vi "All_Combined_final_opt_save_file_P4.vi"() -> ()   [LabVIEW 2018]
uses:
  <vilib>/LabVIEW Interface for Arduino/Type Defs/Board Type.ctl
  Controls created/Control 3.ctl
  Controls created/Control 4.ctl
  <vilib>/LabVIEW Interface for Arduino/Type Defs/Connection Type.ctl
  <instrlib>/LeCroy Wave Series/Public/Data/Read Single Waveform.vi
  <vilib>/Utility/file.llb/Write Delimited Spreadsheet (DBL).vi
  <vilib>/LabVIEW Interface for Arduino/LabVIEW Interface for Arduino.lvlib
  <instrlib>/Siglent SDG X Series/Siglent SDG X Series.lvlib
  <instrlib>/LeCroy Wave Series/LeCroy Wave Series.lvlib
panel:
  in  "Tab Control":enum32{"Page 1", "Page 2", "Page 3"}(tab)
  in  "VISA resource":refnum<visa-resource-name>
  in  "Board Type (Uno)":T1
  in  "Steps for 1 rotation(1600steps)":i16=1600
  in  "Set Speed (Steps/s)":i16=1200 min=0 max=3000 step=50
  out "Steps Remaining? 2":bool
  in  "#Steps":i16
  out "Step Angle":dbl
  in  "Baud Rate":u32=9600
  out "Iteration #":i32
  out "Steps Remaining?":bool
  in  "Total translation distance(in mm)":i16
  out "Error":errorcluster
  in  "#Steps":dbl
  in  "Arbitray Movement":bool
  in  "Stop":bool
  out "Moving?":bool
  out "stop motion":bool
  in  "MOTION":bool
  in  "?":i8(slide) step=2 scale=0.0..2.0
  in  "OK Button":bool
  out "# steps moved":i32
  out "Scan_time":dbl
  out "daq_time":dbl
  out "appended array":dbl[](array[numeric])
  in  "VISA Refnum in":refnum<visa-resource-name>="USB0::0xF4EC::0xEE38::SDG2XCAD2R3765::INSTR"
  in  "Channel (1:Channel 1)":i32(ring)=1 items=["Channel 1"=1, "Channel 2"=2]
  in  "Enable Output (T: Enable)":bool=TRUE
  in  "Amplitude (1.0 Vpp)":dbl=20.0 format="%#.3f"
  in  "Frequency (1000 Hz)":T2=1500000.0 format="%#.6g"
  in  "DC Offset (0.00 V) in":dbl
  in  "Waveform Function (0: Sine) in":u16(ring) items=["Sine", "Square", "Ramp", "DC", "Pulse", "Arb"]
  in  "Phase (0.0 degrees)":dbl=0.002 min=-360.0 max=360.0 format="%#.1g"
  in  "Fall (20 ns)":dbl=8.4e-09 format="%#.3g"
  in  "Duty (20%)":dbl=4.32 min=0.0001 max=100.0 format="%.4g"
  in  "Delay (0.00 s)":dbl min=-1000000.0 max=1000000.0
  in  "Rise (20 ns)":dbl=1.04e-08 format="%#.3g"
  in  "True To \ngenerate\n pulse":T3=TRUE
  out "VISA resource name out":refnum<visa-resource-name>
  out "error out":errorcluster
  out "Output Filename":path
  out "error out 2":errorcluster
  in  "format string":string="Channel: %g \nWavetype: %g \nAMP: %gV\nFreq: %gHz \nRiseTime: %gs \nFallTime: %gs \nDutyCycle: %g"
  out "Output Directory":path
  in  "File Directory":path=path "E:/Ankur/Labview/Automation/Data/Exp1"
  in  "Filename":string
  out "Oscilloscope\n Runnning":bool
  in  "stop":bool
  out "Waveform Data":waveform(dbl)(graph)
  in  "Timeout (10000 ms)":u32=10000
  in  "Source (0: Channel 1)":u16(ring) items=["Channel 1", "Channel 2", "Channel 3", "Channel 4", "Memory 1", "Memory 2", "Memory 3", "Memory 4", "Function 1", "Function 2", "Function 3", "Function 4", "Function 5", "Function 6", "Function 7", "Function 8"]
  in  "Perform Auto Setup?":bool
  in  "Reset Scope?":bool
  in  "VISA resource name":refnum<visa-resource-name>="LecroyHDO4024-1"
  in  "Save Files in Directory (In Oscilloscope)":string="D:\\Automation\\Data"
  in  "Filename":string="Title"
  in  "Path to save DATA":path=path "E:/Ankur/Labview/Automation/Files/Oscdata"
  out "Saved filename":string
  in  "Save File locally":bool
  # "For Rotational motion"
  # "For Translational Motion"
  # "For Translational motion"
  # "OFF"
  # "ON"
  # "Yes"
  # "No"
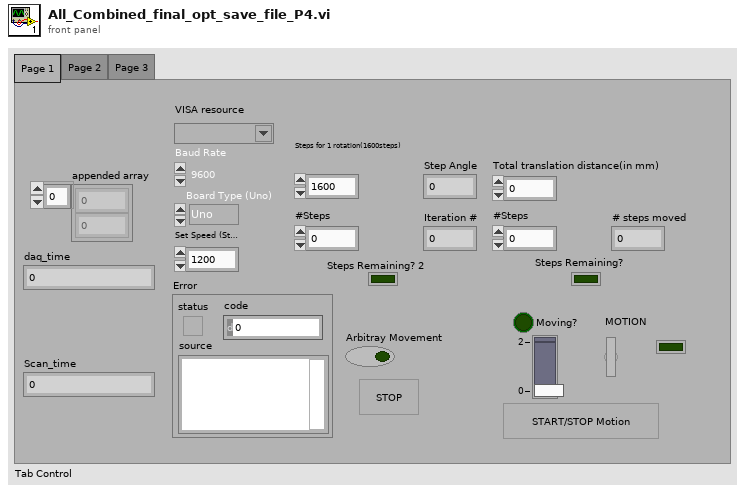
[diagram p1: front panel]
types:
  T1 = typedef "LabVIEW Interface for Arduino.lvlib/Board Type.ctl" = enum16{"Uno", "Dimuelanove w/Atmega 328", "Mega 2560"}
  T2 = typedef "Control 3.ctl" = dbl
  T3 = typedef "Control 4.ctl" = bool
  T4 = typedef "LabVIEW Interface for Arduino.lvlib/Connection Type.ctl" = enum8{"USB / Serial", "XBEE", "BlueSmirf (Bluetooth)"}
  T5 = typedef "LabVIEW Interface for Arduino.lvlib/Arduino Resource.ctl" = cluster{"VISA resource":refnum<visa-resource-name>, "Board Type":T1, "Connection Type":enum8{"USB / Serial"}, "Bytes Per Packet (15)":u8}
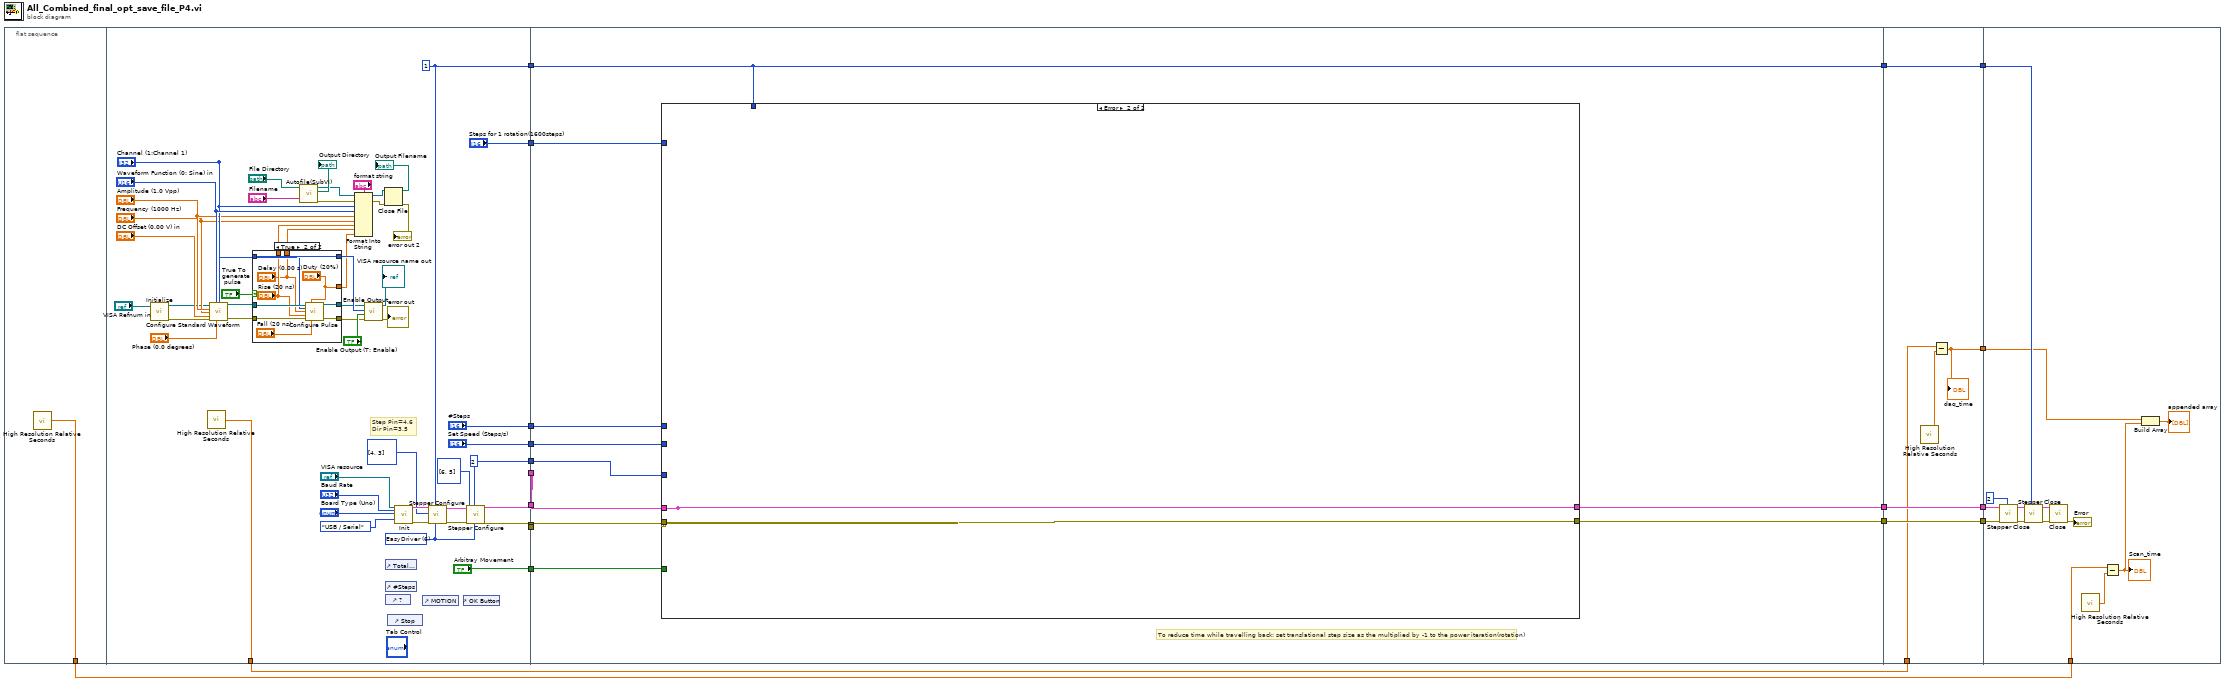
[diagram p0: block diagram]
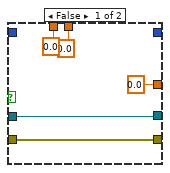
[diagram p2: hidden frame]
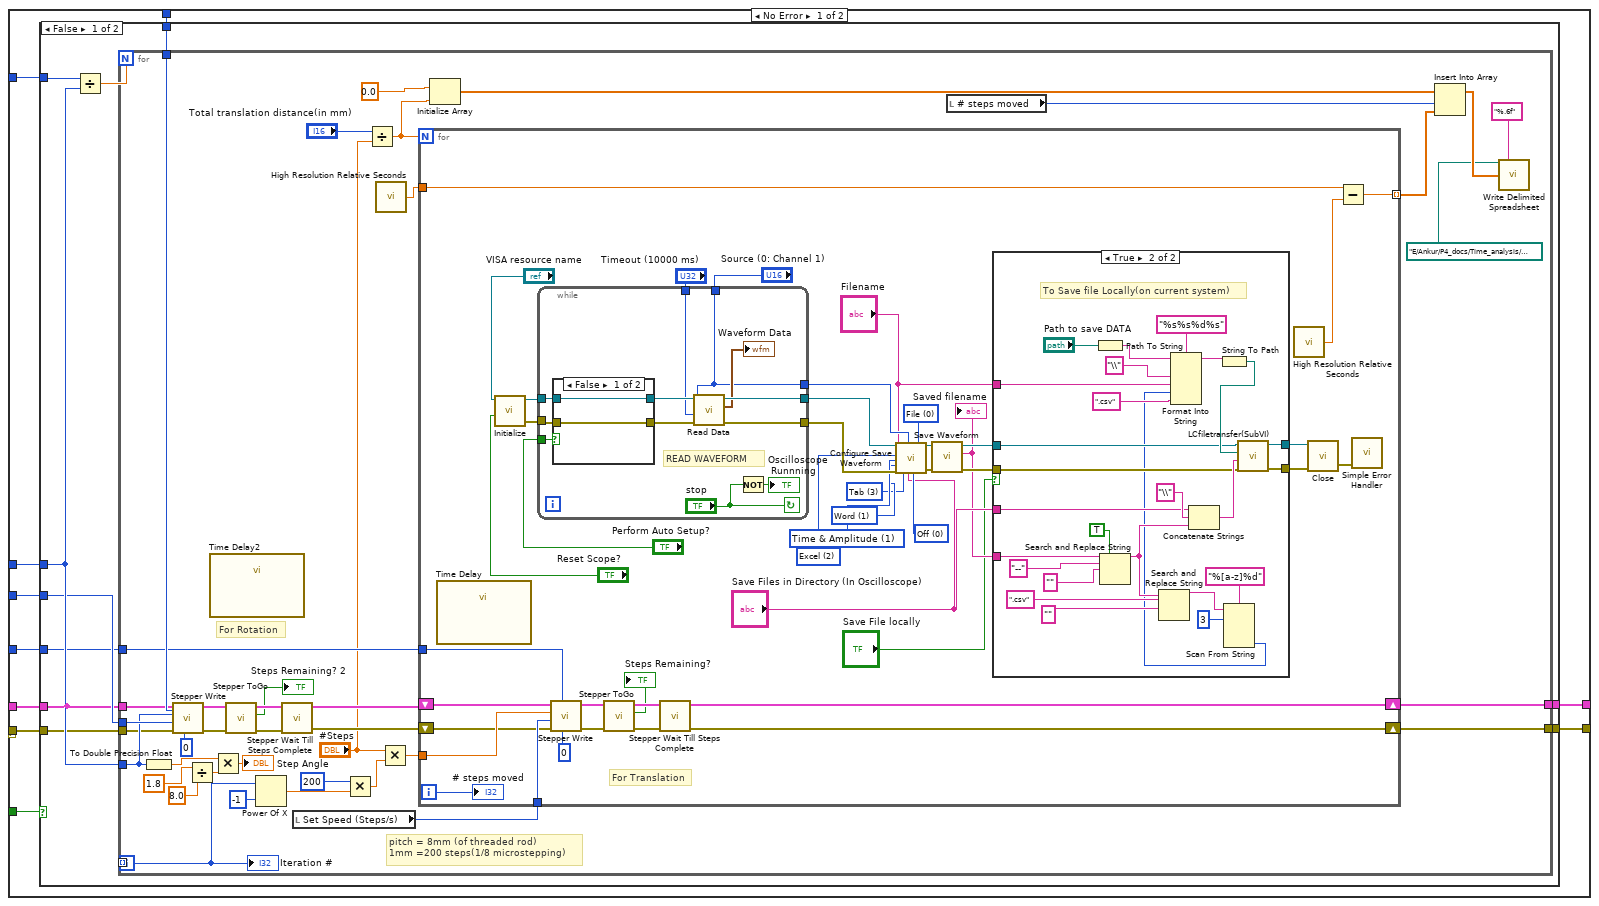
[diagram p3: hidden frame]
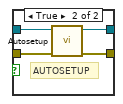
[diagram p5: hidden frame]
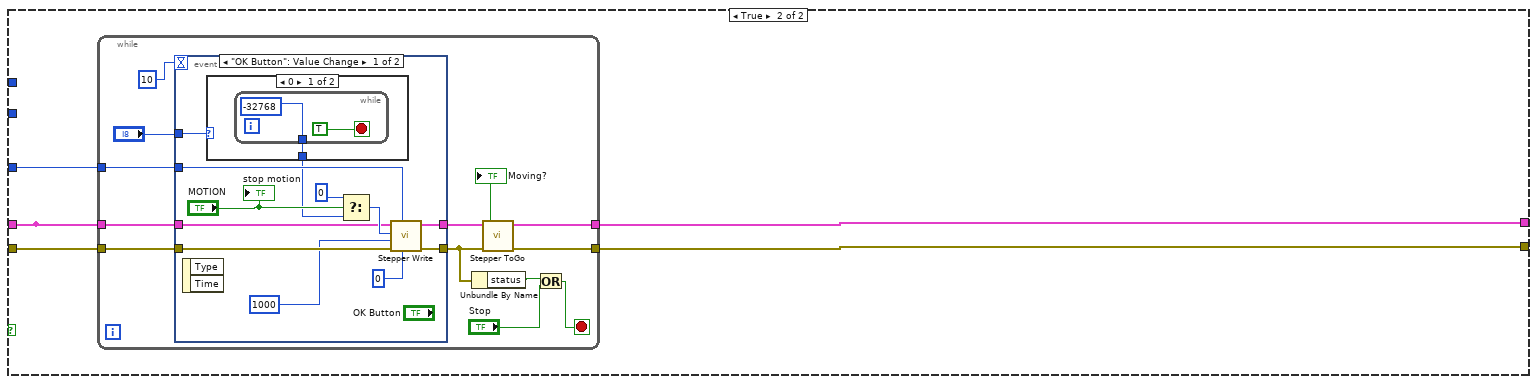
[diagram p6: hidden frame]
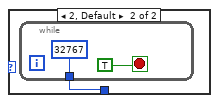
[diagram p7: hidden frame]
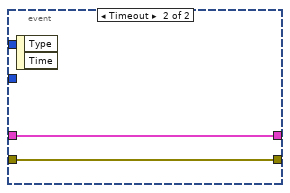
[diagram p8: hidden frame]
diagram:
  n1 = flat-sequence {
    tunnel: [w18] -> w2
    tunnel: [w27] -> w14
    tunnel: [w26] -> w13
    tunnel: [w25] -> w12
    tunnel: [w20] -> w11
    tunnel: ["Arbitray Movement"] -> w10
    tunnel: ["Set Speed (Steps/s)"] -> w9
    tunnel: ["Steps for 1 rotation(1600steps)"] -> w8
    tunnel: ["#Steps"] -> w7
    tunnel: [w19] -> w6
    tunnel: [w89] -> w17
    tunnel: [w92] -> w16
    tunnel: [w91] -> w15
    tunnel: w14 -> [w90]
    tunnel: w13 -> [w89]
    tunnel: w12 -> [w88]
    tunnel: w11 -> [w87]
    tunnel: w10 -> [w86]
    tunnel: w9 -> [w85]
    tunnel: w8 -> [w84]
    tunnel: w7 -> [w83]
    tunnel: w17 -> [w288]
    tunnel: w16 -> [w287]
    tunnel: w15 -> [w286]
    tunnel: w6 -> [w284]
    tunnel: [w288] -> w5
    tunnel: [w287] -> w4
    tunnel: [w286] -> w3
    tunnel: [w283] -> w1
    tunnel: w5 -> [w294]
    tunnel: w4 -> [w296]
    tunnel: w3 -> [w295]
    tunnel: w2 -> [w292]
    tunnel: w1 -> [w291]
    frame #0 {
      n2 = call <vilib>:"High Resolution Relative Seconds.vi"() -> ("relative seconds"=w18:dbl)
    }
    frame #1 {
      w27 = u8 2 ("Stepper #")
      w26 = u8 1 ("Stepper #")
      w31 = u8 6 items=["2 Wire (Pulse & Direction)"=1, "2 Wire"=2, "4 Wire"=4, "EasyDriver"=6, "AF Motor Shield (Stepper 1 & 2 Only)"=5] ("Control Method")
      # "Step Pin=4,6\nDir Pin=3,5"
      n3 = call <instrlib>:"Initialize.vi"("VISA resource name"="VISA Refnum in") -> ("error out"=w44:errorcluster, "VISA resource name out"=w43:refnum<visa-resource-name>)  [unwired: 9 in]
      n4 = call <vilib>:"High Resolution Relative Seconds.vi"() -> ("relative seconds"=w19:dbl)
      n5 = call <instrlib>:"Configure Standard Waveform.vi"("VISA resource name"=w43, "Waveform Function (0: Sine)"="Waveform Function (0: Sine) in", "Channel (1:Channel 1)"="Channel (1:Channel 1)", "Amplitude (1.0 Vpp)"="Amplitude (1.0 Vpp)", "Frequency (1000 Hz)"="Frequency (1000 Hz)", "DC Offset (0.00 V)"="DC Offset (0.00 V) in", "error in (no error)"=w44, "Phase (0.0 degrees)"="Phase (0.0 degrees)") -> ("VISA resource name out"=w48:refnum<visa-resource-name>, "error out"=w45:errorcluster)  [unwired: 6 in]
      n6 = case shown="True" "True To \ngenerate\n pulse" {
        tunnel: [w73 w81] -> w39
        tunnel: [w72 w80] -> w40
        tunnel: w48 -> [w73 w79]
        tunnel: w45 -> [w72 w78]
        tunnel: "Channel (1:Channel 1)" -> [_ w77]
        tunnel: "Channel (1:Channel 1)" -> [_ _]
        tunnel: [0.0 ("Duty (20%)") "Duty (20%)"] -> w52
        tunnel: [0.0 ("Rise (20 ns)") "Rise (20 ns)"] -> w60
        tunnel: [0.0 ("Delay (0.00 s)") "Delay (0.00 s)"] -> w61
        frame False {
        }
        frame True {
          n7 = call <instrlib>:"Configure Pulse.vi"("VISA resource name"=w79, "Duty (20%)"="Duty (20%)", "Channel (1:Channel 1)"=w77, "Delay (0.00 s)"="Delay (0.00 s)", "Rise (20 ns)"="Rise (20 ns)", "error in (no error)"=w78, "Fall (20 ns)"="Fall (20 ns)") -> ("VISA resource name out"=w81:refnum<visa-resource-name>, "error out"=w80:errorcluster)  [unwired: 7 in]
        }
      }
      n8 = call "Autofile(SubVI).vi"("Filename"="Filename", "File Directory"="File Directory") -> ("error out"=w65:errorcluster, "Output Directory"=→"Output Directory":path, "Byte Stream File out"=w64:refnum<file>)  [unwired: 7 in]
      n9 = Format Into String(format string="format string", initial string=w64, error in=w65, "Channel (1:Channel 1)", "Waveform Function (0: Sine) in", "Amplitude (1.0 Vpp)", "Frequency (1000 Hz)", w60, w61, w52) -> (resulting string=w53:refnum<file>, error out=w56:errorcluster)
      n10 = call <instrlib>:"Enable Output.vi"("error in (no error)"=w40, "Enable Output (T: Enable)"="Enable Output (T: Enable)", "Channel (1:Channel 1)"="Channel (1:Channel 1)", "VISA resource name"=w39) -> ("error out"=→"error out":errorcluster, "VISA resource name out"=→"VISA resource name out":refnum<visa-resource-name>)  [unwired: 6 in]
      n11 = Close File(refnum=w53, error in=w56) -> (path=→"Output Filename":path, error out=→"error out 2":errorcluster)
      n12 = control-ref of="?"() -> ()  [unwired: 1 out]
      n13 = control-ref of="Total translation distance(in mm)"() -> ()  [unwired: 1 out]
      n14 = control-ref of="#Steps"() -> ()  [unwired: 1 out]
      n15 = control-ref of="Stop"() -> ()  [unwired: 1 out]
      n16 = call <vilib>:"Init.vi"("VISA resource"="VISA resource", "Baud Rate (115200)"="Baud Rate", "Board Type (Uno)"="Board Type (Uno)", "Connection Type (USB/Serial)"=Connection_Type."USB / Serial") -> ("Arduino Resource"=w34:T5, "error out"=w35:errorcluster)  [unwired: 14 in]
      n17 = control-ref of="MOTION"() -> ()  [unwired: 1 out]
      n18 = call <vilib>:"Stepper Configure.vi"("Control Method"=w31, "Stepper #"=w26, "error in"=w35, "Stepper Pins"=u8[] [4, 3], "Arduino Resource"=w34) -> ("error out"=w38:errorcluster, "Arduino Resource Out"=w37:T5)  [unwired: 5 in]
      n19 = control-ref of="OK Button"() -> ()  [unwired: 1 out]
      n20 = call <vilib>:"Stepper Configure.vi"("Control Method"=w31, "Stepper #"=w27, "error in"=w38, "Stepper Pins"=u8[] [6, 5], "Arduino Resource"=w37) -> ("error out"=w25:errorcluster, "Arduino Resource Out"=w20:T5)  [unwired: 5 in]
    }
    frame #2 {
      # "To reduce time while travelling back: set translational step size as the multiplied by -1 to the power iteration(rotation)"
      n21 = case shown="Error" w88 {
        tunnel: [w96 w281] -> w92
        tunnel: [w103 w282] -> w91
        tunnel: [w102 w282] -> _
        tunnel: w83 -> [w101 _]
        tunnel: w84 -> [w100 _]
        tunnel: w85 -> [w99 _]
        tunnel: w86 -> [w98 _]
        tunnel: w89 -> [w97 _]
        tunnel: w90 -> [w95 _]
        tunnel: w87 -> [w94 w282]
        tunnel: w88 -> [w93 w281]
        frame No Error {
          n22 = case shown="False" w98 {
            tunnel: [w112 w247] -> w103
            tunnel: [w105 w245] -> w102
            tunnel: w101 -> [w110 _]
            tunnel: w100 -> [w109 _]
            tunnel: w99 -> [w108 _]
            tunnel: w97 -> [w107 _]
            tunnel: [w113 w243] -> w96
            tunnel: w95 -> [w106 w246]
            tunnel: w94 -> [w105 w245]
            tunnel: w93 -> [w104 w244]
            frame False {
              n23 = Divide(x=w109, y=w110) -> (x/y=w111:dbl)
              n24 = for {
                N: w111 -> [_]
                tunnel: [w123] -> w113
                tunnel: [w124] -> w112
                tunnel: w108 -> [w149]
                tunnel: [w130] -> _ mode=indexing
                tunnel: w110 -> [w144]
                tunnel: w107 -> [w139]
                tunnel: w106 -> [w138]
                tunnel: w105 -> [w132]
                tunnel: w104 -> [w131]
                i -> [w130]
                # "pitch = 8mm (of threaded rod)\n1mm =200 steps(1/8 microstepping)"
                # "For Rotation"
                n25 = To Double Precision Float(number=w144) -> (double precision float=w145:dbl)
                n26 = call <vilib>:"Stepper Write.vi"("Set Acceleration (0 to disable)"=i16 0 ("Acceleration"), "Stepper #"=w139, "error in"=w131, "Set Speed (Steps per Second)"=w149, "# of Steps to Move"=w144, "Arduino Resource"=w132) -> ("error out"=w148:errorcluster, "Arduino Resource Out"=w147:T5)  [unwired: 4 in]
                n27 = Divide(x=1.8 ("y"), y=8.0) -> (x/y=w134:dbl)
                n28 = call "Time Delay2"() -> ()  [unwired: 11 in, 1 out]
                n29 = Multiply(x=w145, y=w134) -> (x*y=→"Step Angle":dbl)
                n30 = call <vilib>:"Stepper ToGo.vi"("error in"=w148, "Arduino Resource"=w147) -> ("error out"=w152:errorcluster, "Steps Remaining?"=→"Steps Remaining? 2":bool, "Arduino Resource Out"=w151:T5)  [unwired: 6 in, 1 out]
                n31 = Power Of X(1:-1 ("x"), 2:w130) -> (0:w125:dbl)
                n32 = call <vilib>:"Stepper Wait Till Steps Complete.vi"("error in"=w152, "Arduino Resource In"=w151) -> ("error out"=w143:errorcluster, "Arduino Resource Out"=w142:T5)  [unwired: 8 in]
                n33 = local read "Set Speed (Steps/s)"() -> (w141:i16)
                n34 = Multiply(x=i16 200 ("y"), y=w125) -> (x*y=w127:dbl)
                n35 = Divide(x="Total translation distance(in mm)", y="#Steps") -> (x/y=w121:dbl)
                n36 = call <vilib>:"High Resolution Relative Seconds.vi"() -> ("relative seconds"=w122:dbl)
                n37 = Multiply(x="#Steps", y=w127) -> (x*y=w136:dbl)
                n38 = for {
                  N: w121 -> [_]
                  shift-right: [w191] -> w124
                  shift-left: w142 -> [w187]
                  shift-right: [w190] -> w123
                  shift-left: w143 -> [w186]
                  tunnel: w136 -> [w189]
                  tunnel: w141 -> [w188]
                  tunnel: w138 -> [w183]
                  tunnel: w122 -> [w154]
                  tunnel: [w153] -> w117 mode=indexing
                  i -> [w184]
                  w169 = u16 3 items=["Comma", "Space", "Semicolon", "Tab"] ("Delimiter (  0:Comma)")
                  w168 = u16 0 items=["Off", "Wrap", "Fill"] ("Auto Save (0:Off")
                  w170 = u16 1 items=["Byte", "Word", "Auto"] ("BinarySubFormat (1: Word)")
                  w171 = u16 1 items=["Amplitude Only", "Time & Amplitude", "With Header"] ("SubFormat (1: Time & Amplitude)")
                  w172 = u16 2 items=["Binary", "ASCII", "Excel", "MATLAB", "MathCad", "WaveML"] ("Format (0: Binary)")
                  w167 = u16 0 items=["File", "M1", "M2", "M3", "M4"] ("Destination (0:File)")
                  # "For Translation"
                  n39 = call "Time Delay"() -> ()  [unwired: 11 in, 1 out]
                  n40 = call <instrlib>:"Initialize.vi"("Reset? (T: Yes)"="Reset Scope?", "VISA resource name"="VISA resource name") -> ("error out"=w175:errorcluster, "VISA resource name out"=w174:refnum<visa-resource-name>)  [unwired: 8 in]
                  n41 = while {
                    tunnel: [w234] -> w181
                    tunnel: [w233] -> w180
                    tunnel: "Perform Auto Setup?" -> [w232]
                    tunnel: "Source (0: Channel 1)" -> [w225]
                    tunnel: w175 -> [w231]
                    tunnel: w174 -> [w230]
                    tunnel: "Timeout (10000 ms)" -> [w229]
                    tunnel: [w225] -> w182
                    stop <- "stop" continue-if-true
                    # "READ WAVEFORM"
                    n42 = case shown="False" w232 {
                      tunnel: w231 -> [w237 w242]
                      tunnel: w230 -> [w238 w241]
                      tunnel: [w238 w240] -> w236
                      tunnel: [w237 w239] -> w235
                      frame False {
                      }
                      frame True {
                        # "AUTOSETUP"
                        n43 = call <instrlib>:"Autosetup.vi"("error in (no error)"=w242, "VISA resource name"=w241) -> ("error out"=w239:errorcluster, "VISA resource name out"=w240:refnum<visa-resource-name>)  [unwired: 8 in]
                      }
                    }
                    n44 = call-poly <instrlib>:"Read Data.vi"("error in (no error)"=w235, "Timeout (10000 ms)"=w229, "Source (0: Channel 1)"=w225, "VISA resource name"=w236) -> ("error out"=w234:errorcluster, "Waveform Data"=→"Waveform Data":waveform(dbl), "VISA resource name out"=w233:refnum<visa-resource-name>)  [unwired: 5 in]
                    n45 = Not(x="stop") -> (.not. x?=→"Oscilloscope\n Runnning":bool)
                  }
                  n46 = call <vilib>:"Stepper Write.vi"("Set Acceleration (0 to disable)"=i16 0, "Stepper #"=w183, "error in"=w186, "Set Speed (Steps per Second)"=w188, "# of Steps to Move"=w189, "Arduino Resource"=w187) -> ("error out"=w193:errorcluster, "Arduino Resource Out"=w192:T5)  [unwired: 4 in]
                  n47 = call <vilib>:"Stepper ToGo.vi"("error in"=w193, "Arduino Resource"=w192) -> ("error out"=w196:errorcluster, "Steps Remaining?"=→"Steps Remaining?":bool, "Arduino Resource Out"=w195:T5)  [unwired: 6 in, 1 out]
                  n48 = call <vilib>:"Stepper Wait Till Steps Complete.vi"("error in"=w196, "Arduino Resource In"=w195) -> ("error out"=w190:errorcluster, "Arduino Resource Out"=w191:T5)  [unwired: 8 in]
                  n49 = call <instrlib>:"Configure Save Waveform.vi"("VISA resource name"=w180, "Trace Title (Title)"="Filename", "Format (0: Binary)"=w172, "SubFormat (1: Time & Amplitude)"=w171, "BinarySubFormat (1: Word)"=w170, "error in (no error)"=w181, "Delimiter (  0:Comma)"=w169, "Source (0: Channel 1)"=w182, "Save Files in Directory (D:\\Waveforms)"="Save Files in Directory (In Oscilloscope)", "Auto Save (0:Off"=w168, "Destination (0:File)"=w167) -> ("VISA resource name out"=w166:refnum<visa-resource-name>, "error out"=w165:errorcluster)  [unwired: 7 in]
                  n50 = call <instrlib>:"Save Waveform.vi"("error in (no error)"=w165, "VISA resource name"=w166) -> ("error out"=w160:errorcluster, "Saved filename"=w158:string, "VISA resource name out"=w159:refnum<visa-resource-name>)  [unwired: 7 in]
                  "Saved filename" <- w158
                  n51 = case shown="True" "Save File locally" {
                    tunnel: [w198 w221] -> w163
                    tunnel: [w197 w220] -> w162
                    tunnel: "Save Files in Directory (In Oscilloscope)" -> [_ w214]
                    tunnel: w160 -> [w197 w213]
                    tunnel: w159 -> [w198 w212]
                    tunnel: w158 -> [_ w211]
                    tunnel: "Filename" -> [_ w210]
                    frame False {
                    }
                    frame True {
                      # "To Save file Locally(on current system)"
                      n52 = Path To String(path="Path to save DATA") -> (string=w215:string)
                      n53 = Search and Replace String(replace all?=TRUE ("replace all? (F)"), input string=w211, search string="--", replace string="" ("replace string (\"\")")) -> (result string=w206:string)  [unwired: 4 in, 3 out]
                      n54 = Search and Replace String(input string=w206, search string=".csv", replace string="" ("replace string (\"\")")) -> (result string=w209:string)  [unwired: 5 in, 3 out]
                      n55 = Concatenate Strings(w214, "\\" ("string"), w206) -> (w222:string)
                      n56 = Scan From String(format string="%[a-z]%d", input string=w209, initial scan location=u32 3) -> (output 2=w202:i32)  [unwired: 4 in, 3 out]
                      n57 = Format Into String(format string="%s%s%d%s", initial string=w215, "\\" ("input 1"), w210, w202, ".csv" ("input 3")) -> (resulting string=w201:string)  [unwired: 1 in, 1 out]
                      n58 = String To Path(string=w201) -> (path=w219:path)
                      n59 = call <userlib>:"LCfiletransfer(SubVI).vi"("error in (no error)"=w213, "Source Filename"=w222, "file path (use dialog)"=w219, "VISA Refnum in"=w212) -> ("error out"=w220:errorcluster, "VISA Refnum out"=w221:refnum<visa-resource-name>)  [unwired: 5 in, 1 out]
                    }
                  }
                  n60 = call <vilib>:"High Resolution Relative Seconds.vi"() -> ("relative seconds"=w155:dbl)
                  n61 = call <vilib>:"Close.vi"("error in (no error)"=w162, "VISA resource name"=w163) -> ("error out"=w164:errorcluster)  [unwired: 9 in]
                  n62 = Subtract(x=w154, y=w155) -> (x-y=w153:dbl)
                  n63 = call <vilib>:"Simple Error Handler.vi"("error in (no error)"=w164) -> ()  [unwired: 4 in, 5 out]
                  "# steps moved" <- w184
                }
                n64 = Initialize Array(0.0, w121) -> (w120:dbl[])
                n65 = local read "# steps moved"() -> (w118:i32)
                n66 = Insert Into Array(array=w120, index=w118, new element=w117) -> (w116:dbl[])
                n67 = call-poly <vilib>:"Write Delimited Spreadsheet.vi"("file path (dialog if empty)"=path "E:/Ankur/P4_docs/Time_analysis/LabVIEW", "format (%.3f)"="%.6f", "1D data"=w116) -> ()  [unwired: 11 in, 2 out]
                "Iteration #" <- w130
              }
            }
            frame True {
              n68 = while {
                tunnel: [w253] -> w247
                tunnel: w246 -> [w252]
                tunnel: w245 -> [w250]
                tunnel: w244 -> [w249]
                tunnel: [w248] -> w243
                stop <- w259 stop-if-true
                n69 = event shown="[0] \"OK Button\": Value Change" {
                  selector: _ -> [_ _]
                  dyn-events: _ -> [_ _]
                  timeout: 10 -> [_ _]
                  tunnel: [w271 w280] -> w257
                  tunnel: [w272 w279] -> w255
                  tunnel: w252 -> [w267 _]
                  tunnel: "?" -> [w266 _]
                  tunnel: w250 -> [w263 w280]
                  tunnel: w249 -> [w262 w279]
                  event "OK Button": Value Change {
                    n70 = event-data() -> ()  [unwired: 1 in, 2 out]
                    n71 = case shown="0" w266 {
                      tunnel: [w273 w276] -> w264
                      frame 0 {
                        n72 = while {
                          tunnel: [i16 -32768 ("# of Steps to Move")] -> w273
                          stop <- TRUE ("Stop Reverse movement") stop-if-true
                        }
                      }
                      frame 2, Default {
                        n73 = while {
                          tunnel: [i16 32767 ("# of Steps to Move")] -> w276
                          stop <- TRUE ("Stop Forward movement") stop-if-true
                        }
                      }
                    }
                    n74 = Select(t=0, s="MOTION", f=w264) -> (s? t:f=w268:i32)
                    n75 = call <vilib>:"Stepper Write.vi"("Set Acceleration (0 to disable)"=i16 0 ("Set acceleration"), "Stepper #"=w267, "error in"=w262, "Set Speed (Steps per Second)"=i16 1000, "# of Steps to Move"=w268, "Arduino Resource"=w263) -> ("error out"=w272:errorcluster, "Arduino Resource Out"=w271:T5)  [unwired: 4 in]
                    "stop motion" <- "MOTION"
                  }
                  event Timeout {
                    n76 = event-data() -> ()  [unwired: 1 in, 2 out]
                  }
                }
                n77 = Unbundle By Name(w255) -> ("status"=w258:bool)
                n78 = call <vilib>:"Stepper ToGo.vi"("error in"=w255, "Arduino Resource"=w257) -> ("error out"=w248:errorcluster, "Steps Remaining?"=→"Moving?":bool, "Arduino Resource Out"=w253:T5)  [unwired: 6 in, 1 out]
                n79 = Or(x=w258, y="Stop") -> (x .or. y?=w259:bool)
              }
            }
          }
        }
        frame Error {
        }
      }
    }
    frame #3 {
      n80 = call <vilib>:"High Resolution Relative Seconds.vi"() -> ("relative seconds"=w285:dbl)
      n81 = Subtract(x=w284, y=w285) -> (x-y=w283:dbl)
      "daq_time" <- w283
    }
    frame #4 {
      n82 = call <vilib>:"Stepper Close.vi"("Stepper #"=u8 2, "error in"=w296, "Arduino Resource"=w295) -> ("error out"=w301:errorcluster, "Arduino Resource Out"=w302:T5)  [unwired: 7 in]
      n83 = call <vilib>:"Stepper Close.vi"("Stepper #"=w294, "error in"=w301, "Arduino Resource"=w302) -> ("error out"=w299:errorcluster, "Arduino Resource Out"=w300:T5)  [unwired: 7 in]
      n84 = call <vilib>:"Close.vi"("Arduino Resource"=w300, "error in"=w299) -> ("error out"=→"Error":errorcluster)  [unwired: 13 in]
      n85 = call <vilib>:"High Resolution Relative Seconds.vi"() -> ("relative seconds"=w293:dbl)
      n86 = Subtract(x=w292, y=w293) -> (x-y=w290:dbl)
      "Scan_time" <- w290
      n87 = Build Array(w291, w290) -> (→"appended array":dbl[])
    }
  }
